vi "Get Name.vi"(8 "error in (no error)":errorcluster, 11 "System in":refnum<class "System.lvclass">) -> (0 "error out":errorcluster, 2 "Name":string, 3 "System out":refnum<class "System.lvclass">)   [LabVIEW 2013, in "System.lvlib" / "System.lvclass"]
uses:
  System.lvclass
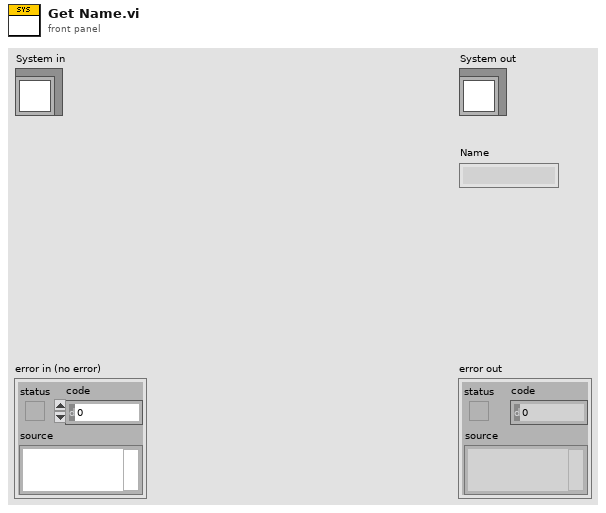
[diagram p1: front panel]
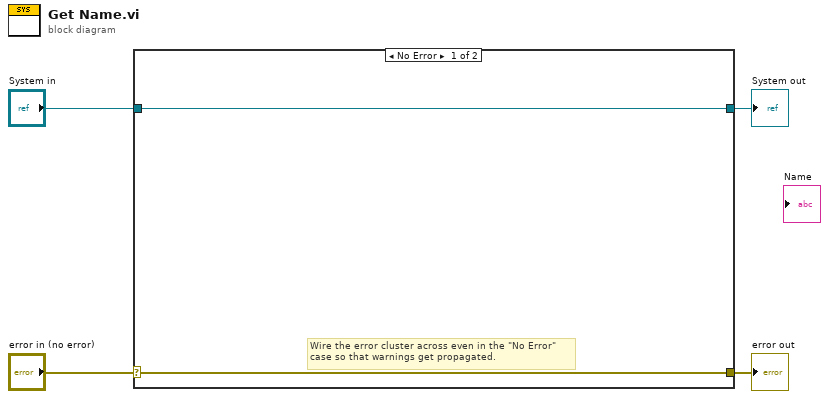
[diagram p0: block diagram]
diagram:
  n1 = case shown="No Error" "error in (no error)" {
    selector: "error in (no error)" -> [w5 w8]
    tunnel: [w5 w8] -> w3
    tunnel: [w6 w7] -> w1
    tunnel: "System in" -> [w6 w7]
    frame No Error {
      # "Wire the error cluster across even in the \"No Error\"\ncase so that warnings get propagated."
    }
    frame Error {
    }
  }
  "error out" <- w3
  "System out" <- w1
